vi "GetErrorBroadcastEvent.vi"(5 "Error In":errorcluster) -> (14 "ErrorBroadcastEvent":refnum<event-registration>, 19 "Error Out":errorcluster)   [LabVIEW 2019, in "Error handler.lvclass"]
uses:
  Error handler.lvclass
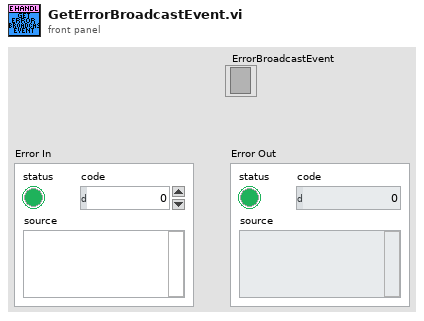
[diagram p1: front panel]
types:
  T1 = typedef "Error handler.lvclass/ObjectAttributes.ctl" = cluster{"ErrorBroadcastEvent":refnum<user-event>, "LoadFPOnError":bool, "ErrorLogFile":refnum<class "ErrorLogFile.lvclass">, "Testing":bool, "Name":string}
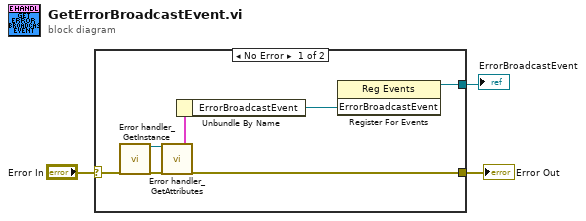
[diagram p0: block diagram]
diagram:
  n1 = case shown="No Error" "Error In" {
    selector: "Error In" -> [w7 w11]
    tunnel: [w9 w11] -> w2
    tunnel: [w4 _] -> w1
    frame No Error {
      n2 = call "Error handler_GetInstance.vi"("error in"=w7) -> ("reference out"=w8:refnum<class "Error handler.lvclass">, "error out"=w6:errorcluster)  [unwired: 14 in, 3 out]
      n3 = call "Error handler_GetAttributes.vi"("reference in"=w8, "error in (no error)"=w6) -> ("Data"=w10:T1, "error out"=w9:errorcluster)  [unwired: 14 in, 2 out]
      n4 = Unbundle By Name(w10) -> ("ErrorBroadcastEvent"=w5:refnum<user-event>)
      n5 = register-events(w5) -> (reference out=w4:refnum<event-registration>)  [unwired: 2 in, 1 out]
    }
    frame Error {
    }
  }
  "Error Out" <- w2
  "ErrorBroadcastEvent" <- w1
